vi "Do_ADAM_channel.vi"(4 "Scan Period":dbl format="%.2f", 5 "Previous Scan Value":dbl format="%.2f", 6 "Present scan array":dbl[](array[numeric]) format="%.2f", 7 "Value to Output":dbl format="%.2f", 8 "Ch Description":T1 {"Duty" format="%.0b"; "D" format="%#_5g"; "C" format="%#_5g"; "B" format="%#_5g"; "A" format="%#_5g"}, 9 "Ch names":string[](array[string])) -> (0 "Scan comment":string, 1 "Output":dbl format="%.3f")   [LabVIEW 2012]
uses:
  ADAM Client/Sub VIs/ADAM Controls/Ch_description_ADAM.ctl
  ADAM Client/Sub VIs/ADAM Controls/Module_type_ADAM.ctl
  ADAM Client/Sub VIs/ADAM Controls/Function_ADAM.ctl
  ADAM Client/Sub VIs/ADAM Controls/Channel_State.ctl
  ADAM Client/Sub VIs/ADAM Controls/Calib_type_ADAM.ctl
  ADAM Client/Sub VIs/ADAM Controls/Address.ctl
  ADAM Serial/Instrument drivers/Arduino/ctls_and_globals/Arduino tx msg cluster.ctl
  ADAM Client/Sub VIs/ADAM Controls/Remember_value_mode.ctl
  ADAM Client/Sub VIs/ADAM Controls/Search_mode.ctl
  Anemometry/Anemometry Sub Vis/Controls/In_Range.ctl
  Anemometry/Anemometry Sub Vis/Globals/Gas_management_global.vi
  ADAM_Global.vi
  Anemometry/Anemometry Sub Vis/Globals/Constants_global.vi
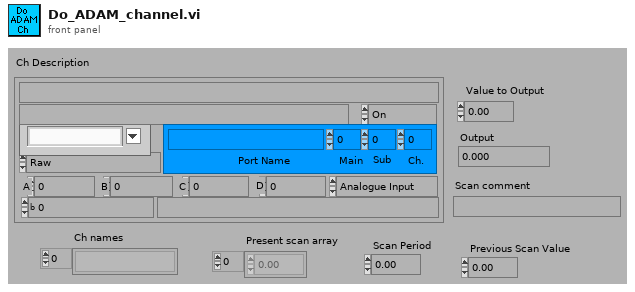
[diagram p1: front panel]
types:
  T1 = typedef "Ch_description_ADAM.ctl" = cluster{"Ch Name":string, "Type":T2, "Function":T3, "Ch State":T4, "Calibration type":T5, "A":dbl, "B":dbl, "C":dbl, "D":dbl, "Comments":string, "Address":T6, "String":string, "Duty":u16}
  T2 = typedef "Module_type_ADAM.ctl" = string
  T3 = typedef "Function_ADAM.ctl" = enum16{"Analogue Input", "Digital Input", "Event counter", "Event rate", "Analogue Output", "Digital Output", "Relay Output"}
  T4 = typedef "Channel_State.ctl" = enum16{"On", "Off", "Always On", "Always Off"}
  T5 = typedef "Calib_type_ADAM.ctl" = enum16{"Raw", "Bx + A", "Cx^2 + Bx + A", "Dx^3 + Cx^2 + Bx + A", "In Band", "Hi-Tec Q", "Hi-Tec M_dot", "Text"}
  T6 = typedef "Address.ctl" = cluster{"Main":i32, "Ch.":i32, "Sub":i32, "Port Name":string}
  T7 = typedef "Remember_value_mode.ctl" = enum16{"Read only", "Read and Write"}
  T8 = typedef "Search_mode.ctl" = enum16{"Between times", "All Times"}
  T9 = typedef "In_Range.ctl" = enum16{"%", "±", "% & ±"}
  T10 = typedef "Arduino tx msg cluster.ctl" = cluster{"dest":u8, "A/D":string, "R/W":string, "chan":u8, "val (float)":sgl}
  T11 = typedef "Valco_valve_ph.ctl" = u16
  T12 = cluster{"Centre Times":dbl[], "Output array":dbl[]}
  T13 = cluster{"Centre Times":dbl[], "Output array":dbl[]}[]
  T14 = typedef "LVDateTimeRec.ctl" = cluster{"fractional second":dbl, "second":i32, "minute":i32, "hour":i32, "day of month":i32, "month":i32, "year":i32, "day of week":i32, "day of year":i32, "DST":i32}
  T15 = typedef "Client_State_Cluster.ctl" = cluster{"Client Name":string, "Traverse level State":T16, "People to Email":string[], "Next Contact Time":dbl}
  T16 = typedef "Traverse_Level_State.ctl" = enum16{"Running", "Complete"}
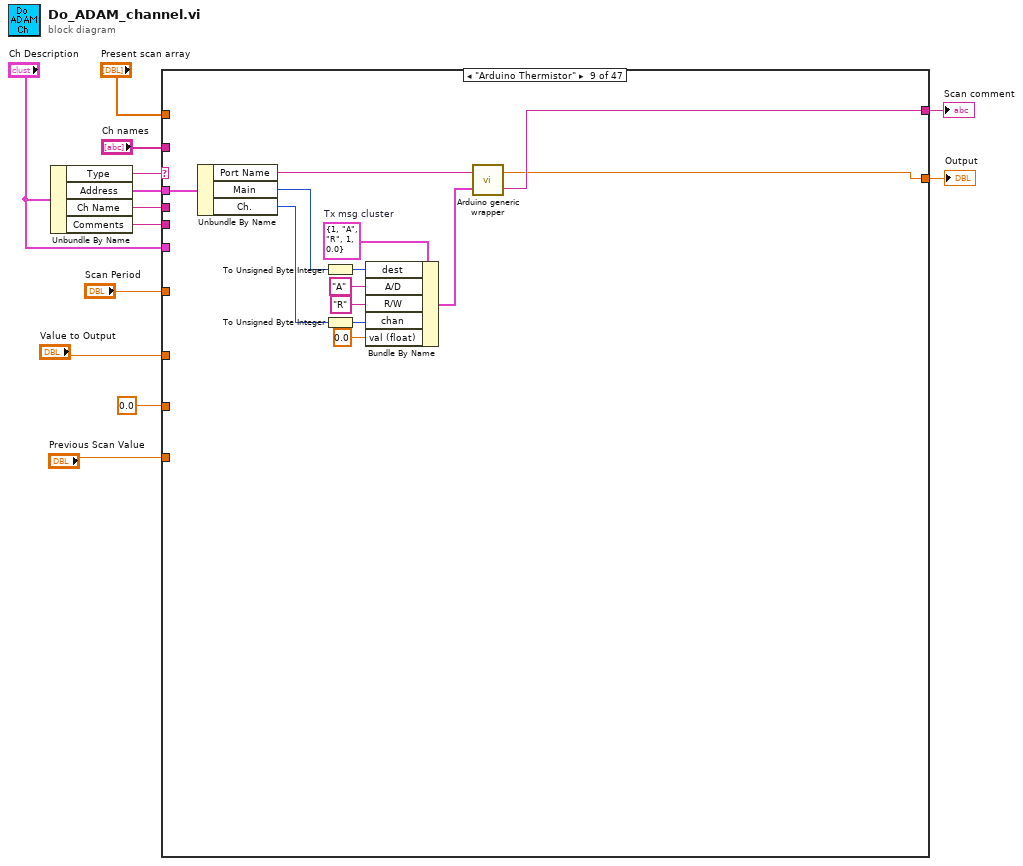
[diagram p0: block diagram]
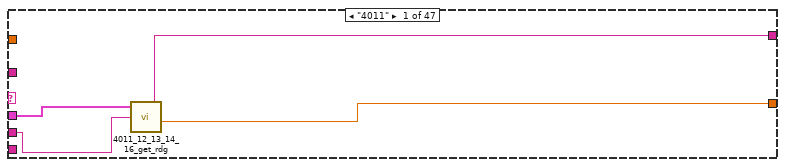
[diagram p2: hidden frame]
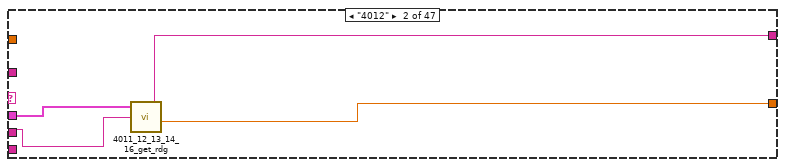
[diagram p3: hidden frame]
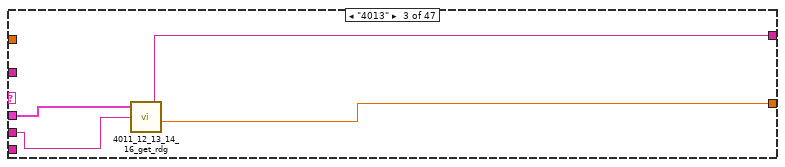
[diagram p4: hidden frame]
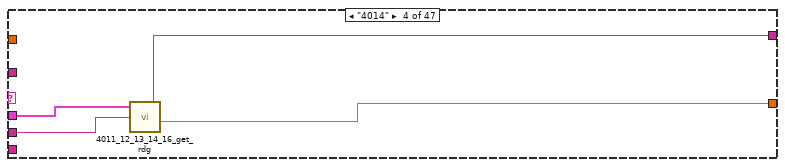
[diagram p5: hidden frame]
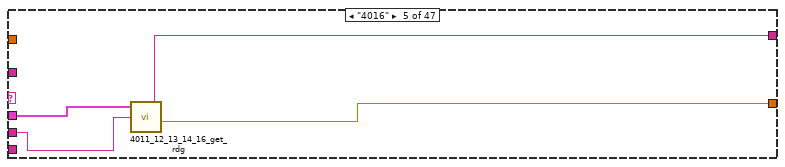
[diagram p6: hidden frame]
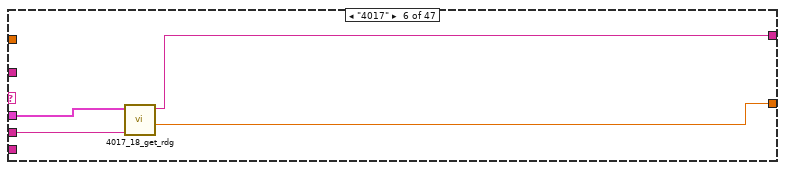
[diagram p7: hidden frame]
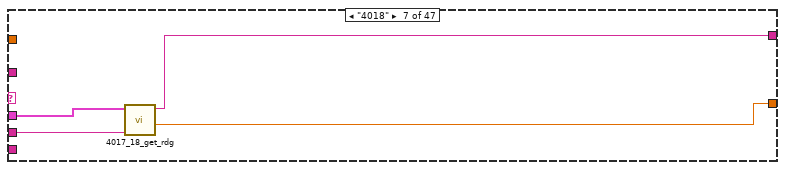
[diagram p8: hidden frame]
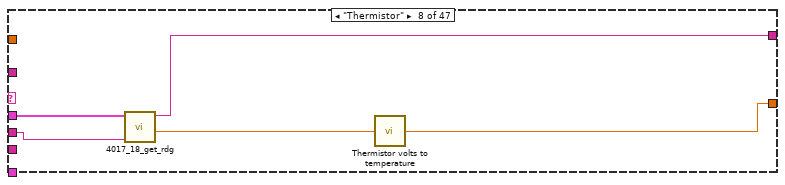
[diagram p9: hidden frame]
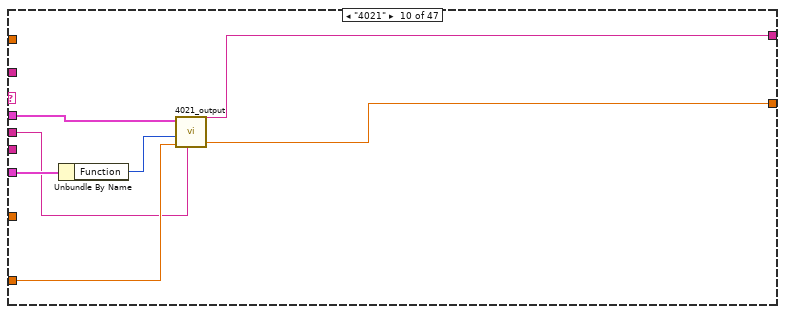
[diagram p10: hidden frame]
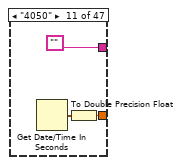
[diagram p11: hidden frame]
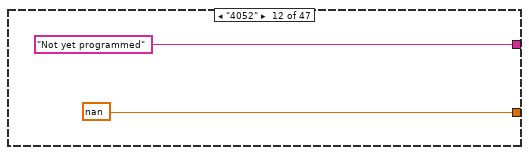
[diagram p12: hidden frame]
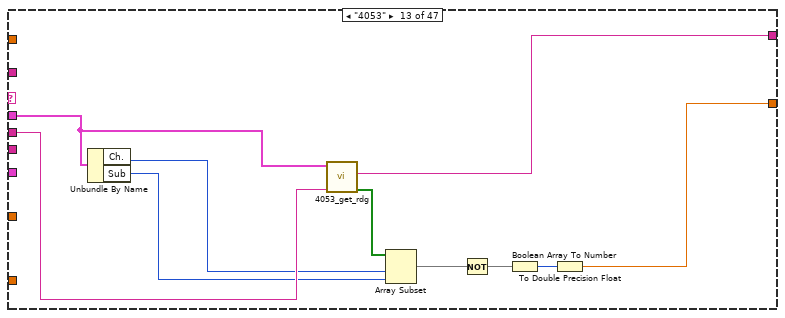
[diagram p13: hidden frame]
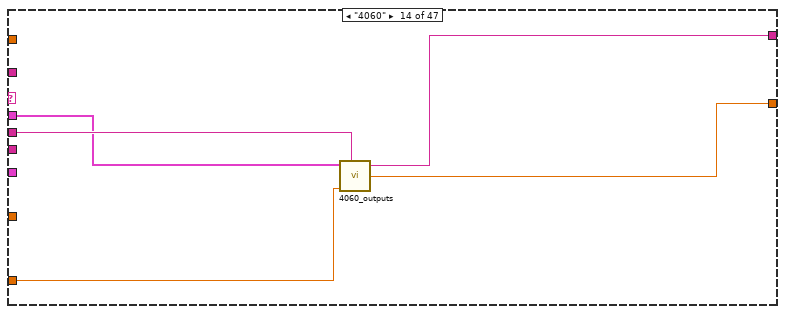
[diagram p14: hidden frame]
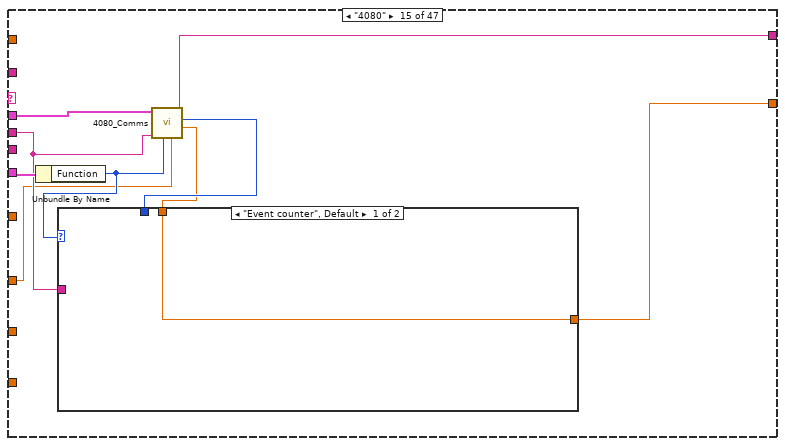
[diagram p15: hidden frame]
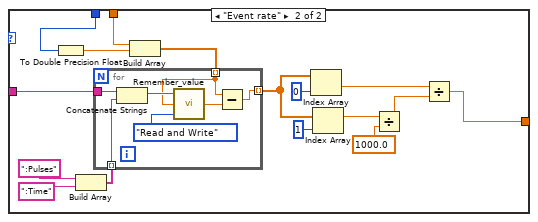
[diagram p16: hidden frame]
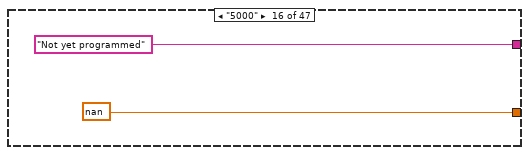
[diagram p17: hidden frame]
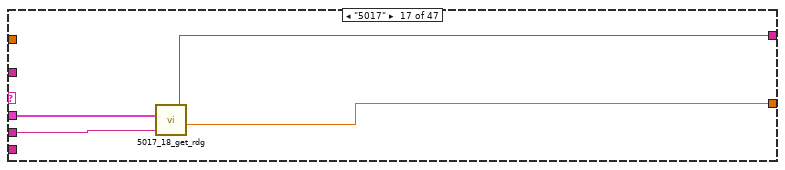
[diagram p18: hidden frame]
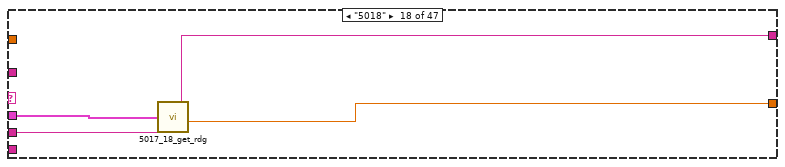
[diagram p19: hidden frame]
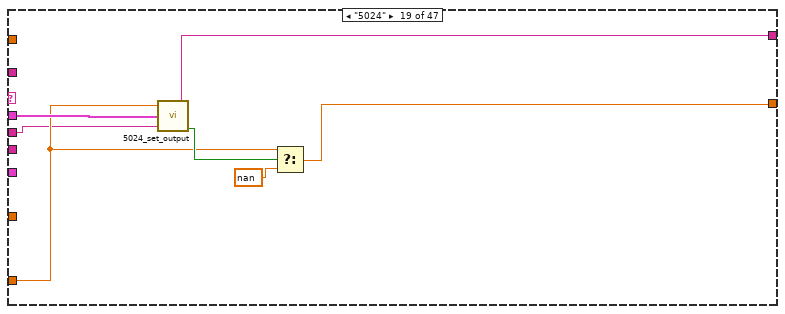
[diagram p20: hidden frame]
diagram:
  n1 = Unbundle By Name("Ch Description") -> ("Type"=w11:T2, "Address"=w10:T6, "Ch Name"=w2:string, "Comments"=w7:string)
  n2 = case shown="\"Arduino Thermistor\"" w11 {
    tunnel: [w16 w20 w24 w28 w32 w36 w40 w42 w47 w65 w68 nan w75 w84 w93 nan w123 w127 w132 w138 w146 w167 w189 w208 nan w276 w278 w294 w317 w356 nan w368 w399 w404 w405 w517 w951 w953 w957 w962 w974 w1008 w1034 w1044 w1049 w1059 0.0 ("Output")] -> w8
    tunnel: [w17 w21 w25 w29 w33 w37 w41 w46 w48 w66 "" "Not yet programmed" w80 w85 w95 "Not yet programmed" w124 w128 w135 w139 w145 w168 w190 w210 "Not yet programmed" w275 w279 w293 w309 w357 "Not yet programmed" w367 w400 w403 w426 w516 "" "" w958 "" "" w997 "" w1045 w1048 "Crazy time based random number!" "Warning; unmatched case in Do_ADAM_channel" ("Status note")] -> w5
    tunnel: w10 -> [w14 w18 w22 w26 w30 w34 w38 w44 w59 w60 _ _ w72 w83 w87 _ w125 w129 w136 w140 w144 w169 w191 w212 _ w273 w277 w296 w314 w362 _ _ w398 w401 _ w508 _ _ _ _ _ _ w1043 w1047 _ _ _]
    tunnel: "Ch Description" -> [_ _ _ _ _ _ _ _ _ w64 _ _ _ _ w94 _ _ _ _ _ w143 w166 w188 w211 _ _ _ _ _ _ _ w373 _ _ w431 w510 _ w954 w959 _ _ _ _ _ w1050 _ _]
    tunnel: w2 -> [w15 w19 w23 w27 w31 w35 w39 w45 _ w61 _ _ w81 w86 w90 _ w122 w126 w130 w137 w141 w163 w185 w209 _ w274 _ w295 w310 w361 _ _ _ w402 _ w513 _ _ _ _ w970 w1004 _ w1046 _ _ _]
    tunnel: "Ch names" -> [_ _ _ _ _ _ _ _ _ _ _ _ _ _ _ _ _ _ _ _ _ _ _ _ _ _ _ _ _ _ _ w374 _ _ w430 w515 _ _ w960 _ _ _ _ _ _ _ _]
    tunnel: "Present scan array" -> [_ _ _ _ _ _ _ _ _ _ _ _ _ _ _ _ _ _ _ _ _ _ _ _ _ _ _ _ _ _ _ w371 _ _ w428 w514 _ _ w961 _ _ _ _ _ _ _ _]
    tunnel: w7 -> [_ _ _ _ _ _ _ _ _ _ _ _ _ _ _ _ _ _ _ _ _ _ _ _ _ _ _ _ _ _ _ w366 _ _ w432 _ _ _ _ _ _ _ _ _ _ _ _]
    tunnel: "Value to Output" -> [_ _ _ _ _ _ _ _ _ w62 _ _ _ w82 w88 _ _ _ w131 _ w142 w164 w186 w207 _ _ _ w292 w318 _ _ w372 _ _ _ _ _ _ _ _ _ _ w1038 _ _ _ _]
    tunnel: "Scan Period" -> [_ _ _ _ _ _ _ _ _ _ _ _ _ _ _ _ _ _ _ _ _ _ _ _ _ _ _ _ _ _ _ w369 _ _ _ w512 _ _ _ _ _ _ _ _ _ _ _]
    tunnel: "Previous Scan Value" -> [_ _ _ _ _ _ _ _ _ _ _ _ _ _ _ _ _ _ _ _ _ _ _ _ _ _ _ _ _ _ _ w370 _ _ w406 w511 w951 _ _ w962 _ _ _ _ _ _ _]
    tunnel: 0.0 -> [_ _ _ _ _ _ _ _ _ _ _ _ _ _ _ _ _ _ _ _ _ _ _ _ _ _ _ _ _ _ _ _ _ _ _ w509 _ _ _ _ _ _ _ _ _ _ _]
    frame "4011" {
      n3 = call "4011_12_13_14_16_get_rdg.vi"("Address"=w14, "Channel Name"=w15) -> ("Comment"=w17:string, "Reading"=w16:dbl)  [unwired: 1 in, 2 out]
    }
    frame "4012" {
      n4 = call "4011_12_13_14_16_get_rdg.vi"("Address"=w18, "Channel Name"=w19) -> ("Comment"=w21:string, "Reading"=w20:dbl)  [unwired: 1 in, 2 out]
    }
    frame "4013" {
      n5 = call "4011_12_13_14_16_get_rdg.vi"("Address"=w22, "Channel Name"=w23) -> ("Comment"=w25:string, "Reading"=w24:dbl)  [unwired: 1 in, 2 out]
    }
    frame "4014" {
      n6 = call "4011_12_13_14_16_get_rdg.vi"("Address"=w26, "Channel Name"=w27) -> ("Comment"=w29:string, "Reading"=w28:dbl)  [unwired: 1 in, 2 out]
    }
    frame "4016" {
      n7 = call "4011_12_13_14_16_get_rdg.vi"("Address"=w30, "Channel Name"=w31) -> ("Comment"=w33:string, "Reading"=w32:dbl)  [unwired: 1 in, 2 out]
    }
    frame "4017" {
      n8 = call "4017_18_get_rdg.vi"("Channel Name"=w35, "Address"=w34) -> ("Reading"=w36:dbl, "Comment"=w37:string)  [unwired: 2 in, 2 out]
    }
    frame "4018" {
      n9 = call "4017_18_get_rdg.vi"("Channel Name"=w39, "Address"=w38) -> ("Reading"=w40:dbl, "Comment"=w41:string)  [unwired: 2 in, 2 out]
    }
    frame "Thermistor" {
      n10 = call "4017_18_get_rdg.vi"("Channel Name"=w45, "Address"=w44) -> ("Reading"=w43:dbl, "Comment"=w46:string)  [unwired: 2 in, 2 out]
      n11 = call "Thermistor volts to temperature.vi"("V2 (V)"=w43) -> ("Temperature (degC)"=w42:dbl)
    }
    frame "Arduino Thermistor" {
      w53 = T10 {"dest"=1, "A/D"="A", "R/W"="R", "chan"=1, "val (float)"=0.0}  # Tx msg cluster
      n12 = Unbundle By Name(w59) -> ("Port Name"=w50:string, "Main"=w51:i32, "Ch."=w52:i32)
      n13 = To Unsigned Byte Integer(number=w51) -> (unsigned 8bit integer=w58:u8)
      n14 = To Unsigned Byte Integer(number=w52) -> (unsigned 8bit integer=w56:u8)
      n15 = Bundle By Name(cluster=w53, "dest"=w58, "A/D"="A", "R/W"="R", "chan"=w56, "val (float)"=sgl 0.0) -> (w49:T10)
      n16 = call "Arduino generic wrapper.vi"("Tx msg cluster"=w49, "Port name"=w50) -> ("Scan comment"=w48:string, "Output"=w47:dbl)
    }
    frame "4021" {
      n17 = Unbundle By Name(w64) -> ("Function"=w63:T3)
      n18 = call "4021_output.vi"("Address"=w60, "Function"=w63, "Set to:"=w62, "Channel Name"=w61) -> ("Comment"=w66:string, "Reading"=w65:dbl)  [unwired: 1 in, 1 out]
    }
    frame "4050" {
      n19 = Get Date/Time In Seconds() -> (seconds since 1Jan1904=w67:timestamp)
      n20 = To Double Precision Float(number=w67) -> (double precision float=w68:dbl)
    }
    frame "4052" {
    }
    frame "4053" {
      n21 = Unbundle By Name(w72) -> ("Ch."=w73:i32, "Sub"=w79:i32)
      n22 = call "4053_get_rdg.vi"("Channel Name"=w81, "Address"=w72) -> ("Boolean array"=w78:bool[], "Comment"=w80:string)  [unwired: 2 in, 2 out]
      n23 = Array Subset(array=w78, index=w73, length=w79) -> (w77:bool[])
      n24 = Not(x=w77) -> (.not. x?=w74:bool[])
      n25 = Boolean Array To Number(Boolean array=w74) -> (number=w76:u32)
      n26 = To Double Precision Float(number=w76) -> (double precision float=w75:dbl)
    }
    frame "4060" {
      n27 = call "4060_outputs.vi"("Address"=w83, "Value to Output"=w82, "Channel Name"=w86) -> ("Comment"=w85:string, "Reading"=w84:dbl)  [unwired: 2 in, 1 out]
    }
    frame "4080" {
      n28 = Unbundle By Name(w94) -> ("Function"=w89:T3)
      n29 = call "4080_Comms.vi"("Value to display"=w88, "Function"=w89, "Channel Name"=w90, "Address"=w87) -> ("Reading"=w91:dbl, "millisecond timer value"=w92:u32, "Comment"=w95:string)  [unwired: 2 in, 1 out]
      n30 = case shown="\"Event counter\", Default" w89 {
        tunnel: w90 -> [_ w112]
        tunnel: w92 -> [_ w105]
        tunnel: [w96 w97] -> w93
        tunnel: w91 -> [w96 w106]
        frame "Event counter", Default {
        }
        frame "Event rate" {
          n31 = To Double Precision Float(number=w105) -> (double precision float=w104:dbl)
          n32 = Build Array(":Pulses", ":Time") -> (w107:string[])
          n33 = Build Array(w106, w104) -> (w103:dbl[])
          n34 = for {
            tunnel: w112 -> [w116]
            tunnel: [w117] -> w100 mode=indexing
            tunnel: w107 -> [w114] mode=indexing
            tunnel: w103 -> [w113] mode=indexing
            n35 = Concatenate Strings(w116, w114) -> (w115:string)
            n36 = call "Remember_value.vi"("Mode"=Remember_value_mode."Read and Write", "Input Value"=w113, "Ch name"=w115) -> ("Output Value"=w118:dbl)
            n37 = Subtract(x=w113, y=w118) -> (x-y=w117:dbl)
          }
          n38 = Index Array(array=w100, index=0) -> (element=w98:dbl)
          n39 = Index Array(array=w100, index=1) -> (element=w99:dbl)
          n40 = Divide(x=w99, y=1000.0) -> (x/y=w110:dbl)
          n41 = Divide(x=w98, y=w110) -> (x/y=w97:dbl)
        }
      }
    }
    frame "5000" {
    }
    frame "5017" {
      n42 = call "5017_18_get_rdg.vi"("Address (all reqd.)"=w125, "Channel Name"=w122) -> ("Comment"=w124:string, "Reading"=w123:dbl)  [unwired: 3 out]
    }
    frame "5018" {
      n43 = call "5017_18_get_rdg.vi"("Address (all reqd.)"=w129, "Channel Name"=w126) -> ("Comment"=w128:string, "Reading"=w127:dbl)  [unwired: 3 out]
    }
    frame "5024" {
      n44 = call "5024_set_output.vi"("Set to:"=w131, "Address (all reqd.)"=w136, "Channel Name"=w130) -> ("Comment"=w135:string, "Good Reply"=w133:bool)  [unwired: 2 out]
      n45 = Select(t=w131, s=w133, f=nan) -> (s? t:f=w132:dbl)
    }
    frame "5051" {
      n46 = call "5051_56_get_inputs.vi"("Address (Main, Sub reqd.)"=w140, "Channel Name"=w137) -> ("Comment"=w139:string, "Single output"=w138:dbl)  [unwired: 3 out]
    }
    frame "5056" {
      n47 = Unbundle By Name(w143) -> ("Function"=w147:T3)
      n48 = case shown="\"Digital Input\"" w147 {
        tunnel: w144 -> [_ w153 w162]
        tunnel: ["This function is not available" w154 w160] -> w145
        tunnel: [nan ("A") w151 w157] -> w146
        tunnel: w142 -> [_ _ w156]
        tunnel: w141 -> [_ w150 w155]
        frame "Analogue Input", Default {
        }
        frame "Digital Input" {
          # "Readback value"
          n49 = call "5060_check_outputs.vi"("Address (Main, Sub reqd.)"=w153, "Channel Name"=w150) -> ("Comment"=w154:string, "Single Channel"=w152:i16)  [unwired: 3 out]
          n50 = To Double Precision Float(number=w152) -> (double precision float=w151:dbl)
        }
        frame "Relay Output" {
          # "Sets single o/p channel"
          n51 = Greater Than 0?(x=w156) -> (x > 0?=w161:bool)
          n52 = call "5056_60_set_single_output.vi"("Channel Name"=w155, "Address (all reqd.)"=w162, "Set state:"=w161) -> ("Comment"=w160:string, "Good Reply"=w159:bool)  [unwired: 2 out]
          n53 = Select(t=w156, s=w159, f=nan) -> (s? t:f=w157:dbl)
        }
      }
    }
    frame "5060" {
      n54 = Unbundle By Name(w166) -> ("Function"=w165:T3)
      n55 = case shown="\"Relay Output\"" w165 {
        tunnel: w169 -> [_ w175 w184]
        tunnel: ["This function is not available" w176 w182] -> w168
        tunnel: [nan ("A") w173 w179] -> w167
        tunnel: w164 -> [_ _ w178]
        tunnel: w163 -> [_ w172 w177]
        frame "Analogue Input", Default {
        }
        frame "Digital Input" {
          # "Readback value"
          n56 = call "5060_check_outputs.vi"("Address (Main, Sub reqd.)"=w175, "Channel Name"=w172) -> ("Comment"=w176:string, "Single Channel"=w174:i16)  [unwired: 3 out]
          n57 = To Double Precision Float(number=w174) -> (double precision float=w173:dbl)
        }
        frame "Relay Output" {
          # "Sets single o/p channel"
          n58 = Greater Than 0?(x=w178) -> (x > 0?=w183:bool)
          n59 = call "5056_60_set_single_output.vi"("Channel Name"=w177, "Address (all reqd.)"=w184, "Set state:"=w183) -> ("Comment"=w182:string, "Good Reply"=w181:bool)  [unwired: 2 out]
          n60 = Select(t=w178, s=w181, f=nan) -> (s? t:f=w179:dbl)
        }
      }
    }
    frame "6060" {
      n61 = Unbundle By Name(w188) -> ("Function"=w187:T3)
      n62 = case shown="\"Digital Input\"" w187 {
        tunnel: w191 -> [_ w197 w206]
        tunnel: ["This function is not available" w198 w204] -> w190
        tunnel: [nan ("A") w195 w201] -> w189
        tunnel: w186 -> [_ _ w200]
        tunnel: w185 -> [_ w194 w199]
        frame "Analogue Input", Default {
        }
        frame "Digital Input" {
          n63 = call "6060_read_all_I-O.vi"("Address (Main, Sub reqd.)"=w197, "Channel Name"=w194) -> ("Comment"=w198:string, "Single Input Channel"=w196:i16)  [unwired: 3 out]
          n64 = To Double Precision Float(number=w196) -> (double precision float=w195:dbl)
        }
        frame "Relay Output" {
          # "Sets single o/p channel"
          n65 = Greater Than 0?(x=w200) -> (x > 0?=w205:bool)
          n66 = call "6060_set_single_output.vi"("Channel Name"=w199, "Address (Main, Ch requd.)"=w206, "Set state:"=w205) -> ("Comment"=w204:string, "Good Reply"=w203:bool)  [unwired: 2 out]
          n67 = Select(t=w200, s=w203, f=nan) -> (s? t:f=w201:dbl)
        }
      }
    }
    frame "Tracker" {
      n68 = while {
        tunnel: w212 -> [w236]
        tunnel: w211 -> [w235]
        tunnel: [w229] -> w210
        tunnel: w209 -> [w228]
        tunnel: [w222] -> w208
        tunnel: w207 -> [w221]
        i -> [w218]
        stop <- w215 continue-if-true
        n69 = Unbundle By Name(w235) -> ("Function"=w234:T3)
        n70 = Unbundle By Name(w236) -> ("Port Name"=w233:string, "Ch."=w224:i32, "Main"=w232:i32, "Sub"=w231:i32)
        n71 = case shown="\"Analogue Output\"" w234 {
          tunnel: [enum16{"Set", "Read"}."Set" ("Set") enum16{"Set", "Read"}."Set" ("Set") enum16{"Set", "Read"}."Set" ("Set") enum16{"Set", "Read"}."Set" ("Set") enum16{"Set", "Read"}."Set" ("Set") enum16{"Set", "Read"}."Read" ("Set") enum16{"Set", "Read"}."Read" ("Set")] -> w219
          tunnel: [enum16{"Logic", "Analogue"}."Analogue" ("Analogue") enum16{"Logic", "Analogue"}."Logic" ("Analogue") enum16{"Logic", "Analogue"}."Logic" ("Analogue") enum16{"Logic", "Analogue"}."Logic" ("Analogue") enum16{"Logic", "Analogue"}."Logic" ("Analogue") enum16{"Logic", "Analogue"}."Logic" ("Analogue") enum16{"Logic", "Analogue"}."Analogue" ("Analogue")] -> w230
          frame "Analogue Output" {
          }
          frame "Digital Output" {
          }
          frame "Relay Output" {
          }
          frame "Event rate" {
          }
          frame "Event counter" {
          }
          frame "Digital Input" {
          }
          frame "Analogue Input" {
          }
        }
        n72 = call "TalkTracker.vi"("PORT NAME"=w233, "Set"=w219, "Channel Name"=w228, "Value to set"=w221, "MODULE ADDRESS"=w232, "LOCATION"=w224, "NO. LOCATIONS"=w231, "Analogue"=w230) -> ("Response"=w226:string, "Good Set?"=w213:bool, "Comment out"=w229:string)  [unwired: 1 in, 4 out]
        n73 = Match Pattern(string=w226, regular expression="\r\n") -> (before substring=w225:string)  [unwired: 4 out]
        n74 = case shown="\"Set\"" w219 {
          tunnel: w225 -> [_ w248]
          tunnel: [w240 w247] -> w223
          tunnel: w221 -> [w242 _]
          tunnel: nan ("Reading") -> [w241 w246]
          tunnel: [w239 w244] -> w216
          tunnel: [0 ("y") 1 ("y")] -> w214
          tunnel: w213 -> [w237 _]
          frame "Set" {
            n75 = Not(x=w237) -> (.not. x?=w239:bool)
            n76 = Select(t=w242, s=w237, f=w241) -> (s? t:f=w240:dbl)
          }
          frame "Read" {
            n77 = String Length(string=w248) -> (length=w250:i32)
            n78 = Fract/Exp String To Number(string=w248, default (0 dbl)=w246) -> (offset past number=w251:i32, number=w249:dbl)  [unwired: 2 out]
            n79 = Equal?(x=w250, y=w251) -> (x = y?=w245:bool)
            n80 = Not(x=w245) -> (.not. x?=w244:bool)
            n81 = Select(t=w249, s=w245, f=w246) -> (s? t:f=w247:dbl)
          }
        }
        n82 = case shown="0, Default" w224 {
          tunnel: w223 -> [w252 w255]
          tunnel: [w252 w253] -> w222
          frame 0, Default {
          }
          frame 283 {
            n83 = Equal To 0?(x=w255) -> (x = 0?=w256:bool)
            n84 = Select(t=nan ("Reading"), s=w256, f=w255) -> (s? t:f=w253:dbl)
          }
        }
        n85 = Less?(x=w218, y=w214) -> (x < y?=w217:bool)
        n86 = And(x=w216, y=w217) -> (x .and. y?=w215:bool)
      }
    }
    frame "WEST" {
    }
    frame "GILL" {
      n87 = call "Gill_get_rdg.vi"("Channel Name"=w274, "Address"=w273) -> ("Output"=w276:dbl, "Status note"=w275:string)  [unwired: 2 in, 2 out]
    }
    frame "ClimatronicsUDP" {
      n88 = call "ClimatronicsUDP_get_rdg.vi"("Address"=w277) -> ("Output"=w278:dbl, "Status note"=w279:string)  [unwired: 5 in]
    }
    frame "JEM" {
      n89 = Unbundle By Name(w296) -> ("Main"=w282:i32, "Ch."=w281:i32, "Port Name"=w291:string)
      n90 = case shown="0, Default" w281 {
        tunnel: [i16[] [-3, -2, -1, 0, 14, 29, 43, 57, 71, 86, 100] i16[] [0, 20, 40, 60, 80, 100, 120]] -> w285
        tunnel: [u8[] [10, 50, 80, 100, 120, 140, 160, 180, 200, 220, 240] u8[] [20, 50, 90, 130, 160, 200, 230]] -> w286
        frame 0, Default {
        }
        frame 1 {
        }
      }
      n91 = Add(x=w282, y=w281) -> (x+y=w280:i32)
      n92 = Threshold 1D Array(2:w292, 3:w285) -> (0:w288:dbl)  [unwired: 1 out]
      n93 = Round To Nearest(number=w288) -> (nearest integer value=w289:dbl)
      n94 = To Long Integer(number=w289) -> (32bit integer=w287:i32)
      n95 = Index Array(array=w286, index=w287) -> (element=w284:u8)
      n96 = call "DMX.vi"("Port Name"=w291, "DMX channel no."=w280, "Set value:"=w284, "Channel Name"=w295) -> ("error"=w290:bool)  [unwired: 2 out]
      n97 = Index Array(array=w285, index=w287) -> (element=w283:i16)
      n98 = case shown="False" w290 {
        tunnel: [w297 nan] -> w294
        tunnel: ["" "Comms Error"] -> w293
        tunnel: w283 -> [w299 _]
        frame False {
          n99 = To Double Precision Float(number=w299) -> (double precision float=w297:dbl)
        }
        frame True {
        }
      }
    }
    frame "VICI" {
      n100 = To Long Integer(number=w318) -> (32bit integer=w313:i32)
      n101 = Unbundle By Name(w314) -> ("Port Name"=w316:string, "Ch."=w315:i32)
      n102 = call "Valco_Valve_Position.vi"("Channel Name"=w310, "Valve Number"=w315, "Port Name"=w316, "Requested Posn."=w313) -> ("Error Message"=w308:string, "Achieved Posn."=w311:T11)  [unwired: 2 out]
      n103 = Empty String/Path?(string/path=w308) -> ()  [unwired: 1 out]
      n104 = case shown="True" TRUE {
        tunnel: w314 -> [w325 _]
        tunnel: w313 -> [w324 _]
        tunnel: [w323 w355] -> w312
        tunnel: w311 -> [_ w355]
        tunnel: w310 -> [w322 _]
        tunnel: [w321 w354] -> w309
        tunnel: w308 -> [_ w354]
        tunnel: w308 -> [w320 _]
        tunnel: "X10" ("Port Name") -> [w319 _]
        frame False {
          n105 = stacked-sequence {
            tunnel: w325 -> [_ _ _ _ _ w346]
            tunnel: w324 -> [_ _ _ _ _ w342]
            tunnel: [_ _ _ _ _ w345] -> w323
            tunnel: w322 -> [_ _ _ _ _ w344]
            tunnel: [_ _ _ _ _ w343] -> w321
            tunnel: w320 -> [_ w331 _ _ _ _]
            tunnel: w319 -> [w326 _ _ w334 _ _]
            frame #0 {
              w328 = 3 items=["-----", "A", "B", "C", "D", "E", "F", "G", "H", "I", "J", "K", "L", "M", "N", "O", "P"] ("House Code")
              n106 = call "X10control.vi"("Port Name"=w326, "Power Request (ON)"=FALSE, "House Code"=w328, "Unit No."=5) -> ()  [unwired: 6 out]
            }
            frame #1 {
              n107 = call "Server_Emails.vi"("Message"=w331, "Contact All clients?"=TRUE, "Subject"="Powering Down FID Valve" ("Error Type")) -> ()  [unwired: 2 in, 3 out]
            }
            frame #2 {
              n108 = Wait (ms)(milliseconds to wait=u32 20000) -> ()  [unwired: 1 out]
            }
            frame #3 {
              w336 = 3 items=["-----", "A", "B", "C", "D", "E", "F", "G", "H", "I", "J", "K", "L", "M", "N", "O", "P"] ("House Code")
              n109 = call "X10control.vi"("Port Name"=w334, "Power Request (ON)"=TRUE, "House Code"=w336, "Unit No."=5) -> ()  [unwired: 6 out]
            }
            frame #4 {
              n110 = Wait (ms)(milliseconds to wait=u32 5000) -> ()  [unwired: 1 out]
            }
            frame #5 {
              n111 = Build Array(1 ("element"), 2 ("element"), w342) -> (w339:i32[])
              n112 = for {
                tunnel: w346 -> [w351]
                tunnel: [w350] -> w345
                tunnel: w344 -> [w349]
                tunnel: [w348] -> w343
                tunnel: w339 -> [w347] mode=indexing
                n113 = Unbundle By Name(w351) -> ("Port Name"=w352:string, "Ch."=w353:i32)
                n114 = call "Valco_Valve_Position.vi"("Channel Name"=w349, "Valve Number"=w353, "Port Name"=w352, "Requested Posn."=w347) -> ("Error Message"=w348:string, "Achieved Posn."=w350:T11)  [unwired: 2 out]
              }
            }
          }
        }
        frame True {
        }
      }
      n115 = To Double Precision Float(number=w312) -> (double precision float=w317:dbl)
    }
    frame "Vaisala" {
      n116 = Unbundle By Name(w362) -> ("Main"=w358:i32, "Ch."=w359:i32, "Port Name"=w360:string)
      n117 = call "HMP231.vi"("Channel Name"=w361, "Port Name"=w360, "Channel"=w359, "Address"=w358) -> ("Output"=w356:dbl, "Status note"=w357:string)  [unwired: 2 out]
    }
    frame "DRUCK" {
    }
    frame "Run VI Named:" {
      n118 = Current VI's Path() -> (path=w383:path)
      n119 = Strip Path(path=w383) -> (stripped path=w384:path)  [unwired: 1 out]
      n120 = call <vilib>:"Trim Whitespace.vi"("string"=w366) -> ("trimmed string"=w365:string)  [unwired: 1 in]
      n121 = Strip Path(path=w384) -> (stripped path=w385:path)  [unwired: 1 out]
      n122 = Build Path(base path=w385, name or relative path="Run_vi_named") -> (appended path=w387:path)
      n123 = Build Path(base path=w387, name or relative path=w365) -> (appended path=w382:path)
      n124 = Open VI Reference(type specifier VI Refnum (for type only)=refnum<vi> refnum, vi path=w382) -> (vi reference=w378:refnum<vi>, error out=w377:errorcluster)  [unwired: 1 in, 3 out]
      n125 = property class="VI Interface Type 0"(reference=w378, error in=w377) -> (reference out=w380:refnum<vi>, error out=w379:errorcluster, "Front Panel Window:Open"=w381:bool)
      n126 = case shown="False" w381 {
        tunnel: w380 -> [w395 w397]
        tunnel: w379 -> [w394 w396]
        tunnel: [w393 w397] -> w376
        tunnel: [w391 w396] -> w375
        frame False {
          n127 = property class="VI Interface Type 0"(reference=w395, error in=w394, "Front Panel Window:Open"=TRUE) -> (reference out=w393:refnum<vi>, error out=w391:errorcluster)
        }
        frame True {
        }
      }
      n128 = call-by-ref "?"(reference=w376, error in=w375, "Scan Period"=w369, "Previous Scan Value"=w370, "Present scan array"=w371, "Value to Output"=w372, "Ch Description"=w373, "Ch names"=w374) -> (reference out=w389:refnum<vi>, error out=w390:errorcluster, "Scan comment"=w367:string, "Output"=w368:dbl)  [unwired: 2 in]
      n129 = Close Reference(reference=w389, error in (no error)=w390) -> ()  [unwired: 1 out]
    }
    frame "IR2100" {
      n130 = call "IR2100_get_rdg.vi"("Address"=w398) -> ("Comment"=w400:string, "Reading"=w399:dbl)  [unwired: 2 in, 2 out]
    }
    frame "PPT" {
      n131 = call "PPT_get_rdg.vi"("Channel Name"=w402, "Address"=w401) -> ("Reading"=w404:dbl, "Comment"=w403:string)  [unwired: 2 in, 2 out]
    }
    frame "Comparator" {
      # "A Warn if above this value\nB Warn if below this value\nC  Hysteresis margin\nD is the averaging time in minutes\nComments   is Channel name to check"
      n132 = Unbundle By Name(w431) -> ("D"=w414:dbl)
      n133 = Match Pattern(string=w432, regular expression=":::" ("String to match")) -> (before substring=w429:string)  [unwired: 4 out]
      n134 = call "Read_value_of_earlier_Ch.vi"("Desired Ch to Read"=w429, "Ch names"=w430, "Present scan array"=w428) -> ("Value"=w413:dbl, "Scan comment"=w427:string)  [unwired: 1 in]
      n135 = Equal?(x=w406, y=1.0) -> (x = y?=w422:bool)
      n136 = Unbundle By Name(w431) -> ("A"=w425:dbl, "B"=w424:dbl, "C"=w423:dbl)
      n137 = Equal To 0?(x=w414) -> (x = 0?=w412:bool)
      n138 = case shown="True" w422 {
        tunnel: [w438 w443] -> w420
        tunnel: w425 -> [w438 w442]
        tunnel: w424 -> [w437 w441]
        tunnel: [w437 w439] -> w421
        tunnel: w423 -> [_ w440]
        frame False {
        }
        frame True {
          n139 = Subtract(x=w442, y=w440) -> (x-y=w443:dbl)
          n140 = Add(x=w441, y=w440) -> (x+y=w439:dbl)
        }
      }
      n141 = case shown="False" w412 {
        tunnel: [w448 w451] -> w435
        tunnel: w429 -> [w450 _]
        tunnel: [w446 w452] -> w411
        tunnel: w414 -> [w444 _]
        tunnel: w413 -> [_ w452]
        tunnel: w427 -> [w448 w451]
        frame False {
          n142 = Build Array(w450) -> (w445:string[])
          n143 = call "Get_Channel_averages.vi"("Desired Ch Names"=w445, "Averaging time (mins)"=w444) -> ("number"=w447:dbl[])  [unwired: 1 in, 2 out]
          n144 = Index Array(array=w447, index=0) -> (element=w446:dbl)
        }
        frame True {
        }
      }
      n145 = Not(x=w422) -> (.not. x?=w415:bool)
      n146 = In Range and Coerce(upper limit=w420, x=w411, lower limit=w421) -> (In Range?=w416:bool)  [unwired: 1 out]
      n147 = Greater?(x=w411, y=w420) -> (0:w419:bool)
      n148 = Not A Number/Path/Refnum?(number/path/refnum=w411) -> (NaN/Path/Refnum?=w408:bool)
      n149 = Equal?(x=w416, y=w415) -> (x = y?=w410:bool)
      n150 = Or(x=w410, y=w408) -> (x .or. y?=w409:bool)
      n151 = case shown="False" w409 {
        tunnel: w429 -> [w459 _]
        tunnel: w420 -> [w458 _]
        tunnel: w431 -> [w457 _]
        tunnel: w421 -> [w456 _]
        tunnel: w416 -> [w455 _]
        tunnel: w411 -> [w454 _]
        tunnel: w419 -> [w453 _]
        frame False {
          n152 = stacked-sequence {
            seq-local: [w465 _ _ _ _] -> [_ _ _ w506 _]
            seq-local: [_ w485 _ _ _] -> [_ _ _ w503 _]
            seq-local: [w463 _ _ _ _] -> [_ _ _ w499 _]
            tunnel: w459 -> [w467 w493 _ w505 _]
            tunnel: w458 -> [w466 _ _ _ _]
            tunnel: w457 -> [_ _ w498 w507 _]
            tunnel: w456 -> [w464 _ _ _ _]
            tunnel: w455 -> [w462 _ _ _ _]
            tunnel: w454 -> [w461 _ _ _ _]
            tunnel: w453 -> [w460 _ _ _ _]
            frame #0 {
              n153 = case shown="True" w462 {
                tunnel: w467 -> [w472 w483]
                tunnel: w466 -> [_ w476]
                tunnel: [w470 w482] -> w465
                tunnel: w464 -> [_ w475]
                tunnel: ["OK " ""] -> w463
                tunnel: w461 -> [w468 _]
                tunnel: w460 -> [_ w473]
                frame True {
                  n154 = Format Into String(format string="The channel named %s is now  %.3f" ("Format String"), w472, w468) -> (resulting string=w470:string)  [unwired: 2 in, 1 out]
                }
                frame False {
                  n155 = Select(t=w476, s=w473, f=w475) -> (s? t:f=w474:dbl)
                  n156 = Select(t="greater", s=w473, f="less") -> (s? t:f=w478:string)
                  n157 = Format Into String(format string="%s is %s than %.3f" ("Format String"), w483, w478, w474) -> (resulting string=w482:string)  [unwired: 2 in, 1 out]
                }
              }
            }
            frame #1 {
              n158 = Build Array(w493) -> (w492:string[])
              n159 = call "Channel_Names_and_indicies.vi"("All Active Channels"=FALSE, "Desired Ch Names"=w492) -> ("Indicies"=w490:i32[])  [unwired: 1 out]
              n160 = call "Specified_Channels_server.vi"("Mode"=Search_mode."All Times", "Requested channels"=w490) -> ("Output array"=w488:dbl[][], "Centre Times"=w484:dbl[])  [unwired: 3 in, 3 out]
              n161 = Index Array(array=w488, index (row)=0) -> (element=w486:dbl[])  [unwired: 1 in]
              n162 = Bundle("Centre Times"=w484, "Output array"=w486) -> (w489:T12)  [unwired: 1 out]
              n163 = Build Array(w489) -> (w485:T13)
            }
            frame #2 {
              w496 = TRUE  # Contact All clients?
              n164 = Unbundle By Name(w498) -> ("String"=w497:string)
              n165 = call "Get_array_values_fr_String.vi"("String Value"=w497) -> ("String array"=w495:string[])  [unwired: 1 out]
              n166 = call "Client_email_addresses.vi"("Extra People to Email"=w495, "Contact All clients?"=w496) -> ()  [unwired: 1 in]
            }
            frame #3 {
              n167 = Unbundle By Name(w507) -> ("Ch Name"=w500:string)
              n168 = Build Array(w505) -> (w504:string[])
              n169 = Concatenate Strings(w499, w500) -> (w501:string)
              n170 = call "Email_Attachment_Plot.vi"("X axis name"="Time", "XY Graph"=w503, "Series Names"=w504, "message"=w506, "subject ([No Subject])"=w501) -> ()  [unwired: 1 in, 1 out]
            }
            frame #4 {
            }
          }
        }
        frame True {
        }
      }
      n171 = Concatenate Strings(w435, "") -> (w426:string)
      n172 = Select(t=0.0, s=w416, f=1.0) -> (s? t:f=w407:dbl)
      n173 = Select(t=w406, s=w408, f=w407) -> (s? t:f=w405:dbl)
    }
    frame "VIRTUAL" {
      n174 = case shown="\"EnFlo_Tunnel:Inlet:K_Factor\"" w513 {
        tunnel: [w527 w541 w555 w577 w592 w603 w619 w650 w677 w712 w716 w750 w801 w827 w854 w874] -> w517
        tunnel: [w518 w547 w553 w581 w586 w601 w628 "" w681 w706 w722 w747 w800 w826 "" w875] -> w516
        tunnel: w515 -> [w524 w549 w559 w583 w588 w606 w630 w654 w683 w708 w724 w748 w806 w831 _ w877]
        tunnel: w514 -> [w525 w548 w560 w582 w587 w607 w629 w655 w684 w707 w723 w749 w808 w833 _ w876]
        tunnel: w513 -> [w522 _ _ _ _ _ _ _ _ _ _ w736 _ _ w849 _]
        tunnel: w512 -> [w523 _ _ _ _ _ _ _ _ _ _ _ w798 w825 w854 w873]
        tunnel: w511 -> [w526 _ _ _ _ _ _ _ _ _ _ w751 w802 w828 _ w872]
        tunnel: w510 -> [_ _ w551 _ _ _ _ _ _ _ _ w742 _ _ _ _]
        tunnel: w509 -> [_ w540 _ _ _ w600 _ _ _ _ _ _ _ _ _ _]
        tunnel: w508 -> [_ _ _ _ _ _ _ _ _ _ _ _ _ _ _ _]
        frame "GMU:Remaining:", Default {
          n175 = Match Pattern(string=w522, regular expression="GMU:Remaining:" ("String to match")) -> (match substring=w520:string)  [unwired: 4 out]
          n176 = Empty String/Path?(string/path=w520) -> (empty?=w519:bool)
          n177 = case shown="False" w519 {
            tunnel: [w534 nan] -> w527
            tunnel: w526 -> [w533 _]
            tunnel: w525 -> [w532 _]
            tunnel: w524 -> [w531 _]
            tunnel: w523 -> [w530 _]
            tunnel: w522 -> [w529 _]
            tunnel: [w528 w536] -> w518
            frame False {
              n178 = call "Update_Rem_gas.vi"("Scan Period (s)"=w530, "Gas Remaining in"=w533, "Ch name"=w529, "Ch names"=w531, "Present scan array"=w532) -> ("Gas Remaining out"=w534:dbl, "Comments"=w528:string)  [unwired: 1 out]
            }
            frame True {
              n179 = Current VI's Path() -> (path=w538:path)
              n180 = Path To String(path=w538) -> (string=w537:string)
              n181 = Concatenate Strings(" was not matched in ", w537) -> (w536:string)
            }
          }
        }
        frame "GMU:Source:Meas Q" {
          n182 = call "Calculate_Release_Flowrates.vi"("Ch names"=w549, "Units"=enum16{"Q l/min", "M_dot Kg/min"}."Q l/min", "Present scan array"=w548) -> ("Trace"=w545:dbl, "Carrier"=w546:dbl, "Scan comments"=w547:string)
          n183 = Add(x=w546, y=w545) -> (x+y=w542:dbl)
          n184 = Not Equal To 0?(x=w542) -> (x != 0?=w543:bool)
          n185 = Select(t=w542, s=w543, f=w540) -> (s? t:f=w541:dbl)
        }
        frame "GMU:Detector:Strength" {
          n186 = Unbundle By Name(w551) -> ("C"=w550:dbl)
          n187 = call "Read_value_of_earlier_Ch.vi"("Desired Ch to Read"="GMU:Detector:Meas Current", "Ch names"=w559, "Present scan array"=w560) -> ("Value"=w556:dbl, "Scan comment"=w554:string)  [unwired: 1 in]
          n188 = Greater?(x=w556, y=w550) -> (0:w557:bool)
          n189 = case shown="True" w557 {
            tunnel: w551 -> [_ w572]
            tunnel: w556 -> [_ w567]
            tunnel: [100.0 ("Eng Values") w565] -> w555
            tunnel: ["Fault" w568] -> w552
            frame False {
            }
            frame True {
              n190 = Unbundle By Name(w572) -> ("D"=w563:dbl, "A"=w571:dbl, "B"=w570:dbl)
              n191 = Less?(x=w567, y=w563) -> (x < y?=w566:bool)
              n192 = Build Array(w571, w570) -> (w569:dbl[])
              n193 = call "Polynomial_convert.vi"("Calib constants"=w569, "Voltage"=w567) -> ("Eng Values"=w564:dbl)  [unwired: 4 out]
              n194 = case shown="True" w566 {
                tunnel: ["Saturated" ""] -> w568
                tunnel: [100.0 ("Eng Values") w575] -> w565
                tunnel: w564 -> [_ w575]
                frame False {
                }
                frame True {
                }
              }
            }
          }
          n195 = Concatenate Strings(w554, w552) -> (w553:string)
        }
        frame "GMU:Source:Meas M_dot" {
          n196 = call "Calculate_Release_Flowrates.vi"("Ch names"=w583, "Units"=enum16{"Q l/min", "M_dot Kg/min"}."M_dot Kg/min", "Present scan array"=w582) -> ("Trace"=w579:dbl, "Carrier"=w580:dbl, "Scan comments"=w581:string)
          n197 = Add(x=w580, y=w579) -> (x+y=w577:dbl)
        }
        frame "GMU:Source:Meas Density" {
          n198 = Build Array("GMU:Source:Meas M_dot", "GMU:Source:Meas Q") -> (w589:string[])
          n199 = call "Read_Earlier_Channels.vi"("Present scan array"=w587, "Ch names"=w588, "Desired Channels"=w589) -> ("Scan comments"=w586:string, "Index 0"=w585:dbl, "Index 1"=w584:dbl)  [unwired: 3 out]
          n200 = Not Equal To 0?(x=w585) -> (x != 0?=w593:bool)
          n201 = case shown="False" w593 {
            tunnel: w585 -> [_ w597]
            tunnel: w584 -> [_ w596]
            tunnel: [0.0 w595] -> w592
            frame False {
            }
            frame True {
              n202 = Divide(x=w597, y=w596) -> (x/y=w598:dbl)
              n203 = Multiply(x=w598, y=1000.0) -> (x*y=w595:dbl)
            }
          }
        }
        frame "GMU:Source:Meas Den Ratio" {
          n204 = call "Read_value_of_earlier_Ch.vi"("Desired Ch to Read"="GMU:Source:Meas Density", "Ch names"=w606, "Present scan array"=w607) -> ("Value"=w602:dbl, "Scan comment"=w601:string)  [unwired: 1 in]
          n205 = Equal?(x=w602, y=w600) -> (x = y?=w604:bool)
          n206 = case shown="False" w604 {
            tunnel: w602 -> [w609 _]
            tunnel: [w608 w614] -> w603
            tunnel: w600 -> [_ w614]
            frame False {
              n207 = global read "Gas_management_global.vi" "Release temp (deg C)"() -> (w612:dbl)
              n208 = global read "Gas_management_global.vi" "Atmos Pres (mbars)"() -> (w611:dbl)
              n209 = call "Gas_Density.vi"("Pressure (mbars)"=w611, "Temperature (deg C)"=w612, "Gas Name"="Air") -> ("Density Kg/m3"=w610:dbl)
              n210 = Divide(x=w609, y=w610) -> (x/y=w608:dbl)
            }
            frame True {
            }
          }
        }
        frame "GMU:Source:Meas Strength" {
          n211 = call "Calculate_Release_Flowrates.vi"("Ch names"=w630, "Units"=enum16{"Q l/min", "M_dot Kg/min"}."Q l/min", "Present scan array"=w629) -> ("Trace"=w622:dbl, "Carrier"=w623:dbl, "Scan comments"=w628:string)
          n212 = Equal To 0?(x=w623) -> (x = 0?=w625:bool)
          n213 = Equal To 0?(x=w622) -> (x = 0?=w626:bool)
          n214 = And(x=w625, y=w626) -> (x .and. y?=w624:bool)
          n215 = case shown="False" w624 {
            tunnel: w623 -> [w641 _]
            tunnel: w622 -> [w640 _]
            tunnel: [w639 0.0] -> w618
            frame False {
              n216 = Add(x=w641, y=w640) -> (x+y=w644:dbl)
              n217 = Divide(x=w640, y=w644) -> (x/y=w643:dbl)
              n218 = Multiply(x=w643, y=100.0) -> (x*y=w639:dbl)
            }
            frame True {
            }
          }
          n219 = while {
            tunnel: [w632] -> w615
            tunnel: [w633] -> w617
            tunnel: w618 -> [w638]
            shift-left: _ -> [w632]
            shift-left: _ -> [w637]
            shift-right: [w638] -> _
            stop <- FALSE continue-if-true
            w636 = 6.0 ("y")
            n220 = Less?(x=w637, y=w636) -> (x < y?=w635:bool)
            n221 = Less?(x=w632, y=w636) -> (x < y?=w634:bool)
            n222 = Or(x=w635, y=w634) -> (x .or. y?=w633:bool)
          }
          n223 = Greater?(x=w618, y=7.0) -> (0:w616:bool)
          n224 = And(x=w617, y=w616) -> (x .and. y?=w620:bool)
          n225 = Select(t=w615, s=w620, f=w618) -> (s? t:f=w619:dbl)
        }
        frame "EnFlo_Tunnel:Temp:Inlet_Av" {
          w653 = 0.0 ("Value")
          w647 = "EnFlo_Tunnel:Temp:Inlet"
          n226 = String Length(string=w647) -> (length=w648:i32)
          n227 = for {
            tunnel: w655 -> [w661] mode=indexing
            tunnel: w654 -> [w660] mode=indexing
            shift-right: [w668] -> w652
            shift-left: w653 -> [w667]
            shift-right: [w665] -> w651
            shift-left: w653 -> [w666]
            tunnel: w648 -> [w664]
            tunnel: w647 -> [w662]
            tunnel: "EnFlo_Tunnel:Temp:Inlet_Av" -> [w659]
            n228 = String Subset(string=w660, length (rest)=w664) -> (substring=w663:string)  [unwired: 1 out]
            n229 = Equal?(x=w663, y=w662) -> (x = y?=w657:bool)
            n230 = Not Equal?(x=w660, y=w659) -> (x != y?=w658:bool)
            n231 = And(x=w657, y=w658) -> (x .and. y?=w656:bool)
            n232 = case shown="True" w656 {
              tunnel: [w670 w674] -> w668
              tunnel: w667 -> [w670 w675]
              tunnel: w661 -> [_ w673]
              tunnel: w666 -> [w669 w672]
              tunnel: [w669 w671] -> w665
              frame False {
              }
              frame True {
                n233 = Add(x=w673, y=w675) -> (x+y=w674:dbl)
                n234 = Increment(x=w672) -> (x+1=w671:dbl)
              }
            }
          }
          n235 = Divide(x=w652, y=w651) -> (x/y=w650:dbl)
        }
        frame "EnFlo Lab:labstrat1:Av Temp" {
          w680 = 0.0 ("Value")
          n236 = for {
            tunnel: w684 -> [w696]
            tunnel: w683 -> [w695]
            shift-right: [w692] -> w681
            shift-left: "" -> [w693]
            shift-right: [w690] -> w679
            shift-left: w680 -> [w689]
            shift-right: [w686] -> w678
            shift-left: w680 -> [w687]
            tunnel: string[] ["EnFlo Lab:labstrat1:Z=4.5m", "EnFlo Lab:labstrat1:Z=3.5m", "EnFlo Lab:labstrat1:Z=2.5m", "EnFlo Lab:labstrat1:Z=1.5m", "EnFlo Lab:labstrat1:Z=0.5m"] -> [w685] mode=indexing
            n237 = call "Read_value_of_earlier_Ch.vi"("Desired Ch to Read"=w685, "Ch names"=w695, "Present scan array"=w696) -> ("Value"=w688:dbl, "Scan comment"=w694:string)  [unwired: 1 in]
            n238 = Concatenate Strings(w693, w694) -> (w692:string)
            n239 = Not A Number/Path/Refnum?(number/path/refnum=w688) -> (NaN/Path/Refnum?=w691:bool)
            n240 = case shown="True" w691 {
              tunnel: [w700 w703] -> w690
              tunnel: w689 -> [w701 w703]
              tunnel: w688 -> [w699 _]
              tunnel: w687 -> [w698 w702]
              tunnel: [w697 w702] -> w686
              frame False {
                n241 = Add(x=w699, y=w701) -> (x+y=w700:dbl)
                n242 = Increment(x=w698) -> (x+1=w697:dbl)
              }
              frame True {
              }
            }
          }
          n243 = Divide(x=w679, y=w678) -> (x/y=w677:dbl)
        }
        frame "EnFlo Lab:labstrat1:Delta T" {
          n244 = Build Array("EnFlo Lab:labstrat1:Z=4.5m", "EnFlo Lab:labstrat1:Z=0.5m") -> (w711:string[])
          n245 = call "Read_Earlier_Channels.vi"("Present scan array"=w707, "Ch names"=w708, "Desired Channels"=w711) -> ("Scan comments"=w706:string, "Index 0"=w705:dbl, "Index 1"=w704:dbl)  [unwired: 3 out]
          n246 = Subtract(x=w705, y=w704) -> (x-y=w712:dbl)
        }
        frame "EnFlo_Tunnel:Inlet:K_Factor" {
          n247 = Build Array("EnFlo_Tunnel:Pressure:Static", "EnFlo_Tunnel:Reference:Velocity", "Froude:NPL:Atmos_Press", "EnFlo_Tunnel:Temp:Inlet_Av") -> (w727:string[])
          n248 = call "Read_Earlier_Channels.vi"("Present scan array"=w723, "Ch names"=w724, "Desired Channels"=w727) -> ("Scan comments"=w722:string, "Index 0"=w717:dbl, "Index 1"=w714:dbl, "Index 2"=w718:dbl, "Index 3"=w719:dbl)  [unwired: 1 out]
          n249 = Greater?(x=w714, y=0.8) -> (0:w715:bool)
          n250 = case shown="True" w715 {
            tunnel: w719 -> [_ w733]
            tunnel: w718 -> [_ w732]
            tunnel: w714 -> [_ w731]
            tunnel: w717 -> [_ w730]
            tunnel: [nan w729] -> w716
            frame False {
            }
            frame True {
              n251 = formula code="Rho=(Patmos*100)/(287*(T+273));\nDyn_Pres=0.5*Rho*U*U;\nK=(-Pstatic/Dyn_Pres)-1;"("Pstatic"=w730, "Patmos"=w732, "T"=w733, "U"=w731) -> ("K"=w729:dbl)  [unwired: 2 out]
            }
          }
        }
        frame "EnFlo_Tunnel:Chilled Water:Valve Dem Pos" {
          n252 = Get Date/Time In Seconds() -> (seconds since 1Jan1904=w735:timestamp)
          n253 = Concatenate Strings(w736, " last updated") -> (w744:string)
          n254 = To Double Precision Float(number=w735) -> (double precision float=w734:dbl)
          n255 = Unbundle By Name(w742) -> ("A"=w741:dbl)
          n256 = call "Remember_value.vi"("Mode"=Remember_value_mode."Read only", "Ch name"=w744) -> ("Output Value"=w743:dbl)  [unwired: 1 in]
          n257 = Subtract(x=w734, y=w743) -> (x-y=w740:dbl)
          n258 = Greater?(x=w740, y=w741) -> (0:w739:bool)
          n259 = Not A Number/Path/Refnum?(number/path/refnum=w740) -> (NaN/Path/Refnum?=w738:bool)
          n260 = Or(x=w738, y=w739) -> (x .or. y?=w737:bool)
          n261 = case shown="True" w737 {
            tunnel: w751 -> [w752 _]
            tunnel: [w752 w770] -> w750
            tunnel: w749 -> [_ w762]
            tunnel: w748 -> [_ w763]
            tunnel: ["" w768] -> w747
            tunnel: w744 -> [_ w758]
            tunnel: w734 -> [_ w754]
            frame False {
            }
            frame True {
              n262 = call "Read_value_of_earlier_Ch.vi"("Desired Ch to Read"="EnFlo_Tunnel:Chiller_Pump:Enable", "Ch names"=w763, "Present scan array"=w762) -> ("Value"=w761:dbl)  [unwired: 1 in, 1 out]
              n263 = Build Array("EnFlo_Tunnel:Chilled Water:Dem Temp", "EnFlo_Tunnel:Chilled Water:Supply", "EnFlo_Tunnel:Chiller_Pump:Running") -> (w769:string[])
              n264 = call "Read_Earlier_Channels.vi"("Present scan array"=w762, "Ch names"=w763, "Desired Channels"=w769) -> ("Scan comments"=w768:string, "Index 0"=w767:dbl, "Index 1"=w766:dbl, "Index 2"=w756:dbl)  [unwired: 2 out]
              n265 = Greater?(x=w761, y=0.5) -> (0:w759:bool)
              n266 = Greater?(x=w756, y=0.5) -> (0:w755:bool)
              n267 = case shown="True" w755 {
                tunnel: [w785 w792] -> w770
                tunnel: w767 -> [_ w794]
                tunnel: w766 -> [_ w793]
                tunnel: w754 -> [_ w791]
                tunnel: w759 -> [w776 _]
                tunnel: w758 -> [_ w790]
                frame False {
                  n268 = Seconds To Date/Time() -> (date time rec=w773:T14)  [unwired: 2 out]
                  n269 = Unbundle By Name(w773) -> ("day of week"=w780:i32, "hour"=w782:i32)
                  n270 = Less?(x=w782, y=3) -> (x < y?=w777:bool)
                  n271 = Equal?(x=7, y=w780) -> (x = y?=w778:bool)
                  n272 = And(x=w778, y=w777) -> (x .and. y?=w775:bool)
                  n273 = case shown="True" w776 {
                    tunnel: w775 -> [w786 w788]
                    tunnel: [w786 w787] -> w774
                    frame False {
                    }
                    frame True {
                      n274 = Not(x=w788) -> (.not. x?=w787:bool)
                    }
                  }
                  n275 = Select(t=0.0, s=w774, f=100.0) -> (s? t:f=w785:dbl)
                }
                frame True {
                  w796 = 100.0  # Max
                  w797 = 0.0  # Min
                  n276 = call "PID.vi"("Present Value"=w793, "Setpoint"=w794) -> ("Dem Output"=w795:dbl)  [unwired: 1 in]
                  n277 = In Range and Coerce(upper limit=w796, x=w795, lower limit=w797) -> (coerced(x)=w792:dbl)  [unwired: 1 out]
                  n278 = call "Remember_value.vi"("Mode"=Remember_value_mode."Read and Write", "Input Value"=w791, "Ch name"=w790) -> ()  [unwired: 1 out]
                }
              }
            }
          }
        }
        frame "EnFlo_Tunnel:Hydrosonic:Integral" {
          n279 = Build Array("EnFlo_Tunnel:Usonic Fixed:Velocity", "Hydrosonic:Transducer:Setting") -> (w807:string[])
          n280 = call "Read_Earlier_Channels.vi"("Present scan array"=w808, "Ch names"=w806, "Desired Channels"=w807) -> ("Scan comments"=w800:string, "Index 0"=w805:dbl, "Index 1"=w799:dbl)  [unwired: 3 out]
          n281 = Greater?(x=w805, y=0.5) -> (0:w803:bool)
          n282 = case shown="True" w803 {
            tunnel: w802 -> [w811 w819]
            tunnel: [w811 w818] -> w801
            tunnel: w799 -> [_ w817]
            tunnel: w798 -> [_ w816]
            frame False {
            }
            frame True {
              w814 = 8640000.0  # Seconds per day x 100
              n283 = Multiply(x=w817, y=w816) -> (x*y=w815:dbl)
              n284 = Divide(x=w815, y=w814) -> (x/y=w813:dbl)
              n285 = Not A Number/Path/Refnum?(number/path/refnum=w813) -> (NaN/Path/Refnum?=w812:bool)
              n286 = case shown="False" w812 {
                tunnel: w819 -> [w822 w823]
                tunnel: [w821 w823] -> w818
                tunnel: w813 -> [w820 _]
                frame False {
                  n287 = Add(x=w820, y=w822) -> (x+y=w821:dbl)
                }
                frame True {
                }
              }
            }
          }
        }
        frame "EnFlo_Tunnel:Days Run at:2.5m/s" {
          n288 = Build Array("EnFlo_Tunnel:Usonic Fixed:Velocity") -> (w832:string[])
          n289 = call "Read_Earlier_Channels.vi"("Present scan array"=w833, "Ch names"=w831, "Desired Channels"=w832) -> ("Scan comments"=w826:string, "Index 0"=w824:dbl)  [unwired: 4 out]
          n290 = Greater?(x=w824, y=0.5) -> (0:w829:bool)
          n291 = case shown="True" w829 {
            tunnel: w828 -> [w835 w843]
            tunnel: [w835 w842] -> w827
            tunnel: w824 -> [_ w841]
            tunnel: w825 -> [_ w840]
            frame False {
            }
            frame True {
              w838 = 216000.0  # Seconds per day x 2.5
              n292 = Multiply(x=w841, y=w840) -> (x*y=w839:dbl)
              n293 = Divide(x=w839, y=w838) -> (x/y=w837:dbl)
              n294 = Not A Number/Path/Refnum?(number/path/refnum=w837) -> (NaN/Path/Refnum?=w836:bool)
              n295 = case shown="True" w836 {
                tunnel: w843 -> [w846 w847]
                tunnel: [w845 w847] -> w842
                tunnel: w837 -> [w844 _]
                frame False {
                  n296 = Add(x=w844, y=w846) -> (x+y=w845:dbl)
                }
                frame True {
                }
              }
            }
          }
        }
        frame "Complete:Scan:Period" {
          n297 = while {
            tunnel: [w857] -> w850
            tunnel: [w864] -> w852
            shift-left: _ -> [w864]
            shift-right: [w865] -> w853
            tunnel: w849 -> [w861]
            tunnel: [w856] -> w848
            stop <- FALSE continue-if-true
            w856 = 10.0 ("Averaging time (mins)")
            n298 = Build Array(w861) -> (w860:string[])
            n299 = call "Get_Channel_averages.vi"("Desired Ch Names"=w860, "Averaging time (mins)"=w856) -> ("number"=w859:dbl[])  [unwired: 1 in, 2 out]
            n300 = Index Array(array=w859, index=0) -> (element=w857:dbl)
            n301 = Greater?(x=w857, y=20.0) -> (0:w865:bool)
          }
          n302 = Compound Arithmetic op=AND(w853, invert w852) -> (w851:bool)
          n303 = case shown="True" w851 {
            tunnel: w850 -> [_ w871]
            tunnel: w848 -> [_ w866]
            frame False {
            }
            frame True {
              n304 = Format Into String(format string="Warning! The average scan period on the ADAM Scan table is %.1f seconds over the last %d minutes." ("Format String"), w871, w866) -> (resulting string=w869:string)  [unwired: 2 in, 1 out]
              n305 = call "Server_Emails.vi"("Message"=w869, "Contact All clients?"=TRUE, "Subject"="Scan Period") -> ()  [unwired: 2 in, 3 out]
            }
          }
        }
        frame "GMU:Source:Est Time" {
          # "NaN's"
          # "Est?"
          # "Inband?"
          n306 = stacked-sequence {
            seq-local: [w878 _ _ _] -> [_ _ w925 _]
            seq-local: [_ w890 _ _] -> [_ _ w922 _]
            seq-local: [_ w891 _ _] -> [_ _ w920 _]
            seq-local: [_ _ w927 _] -> [_ _ _ w943]
            seq-local: [w882 _ _ _] -> [_ _ w924 _]
            seq-local: [_ w889 _ _] -> [_ _ _ w939]
            tunnel: w877 -> [w884 w892 w930 _]
            tunnel: w876 -> [w883 w893 w931 _]
            tunnel: [_ _ w923 _] -> w875
            tunnel: [_ _ _ w942] -> w874
            tunnel: w873 -> [_ _ _ w941]
            tunnel: w872 -> [_ _ _ w940]
            frame #0 {
              n307 = Build Array("GMU:Source:Density Ratio", "GMU:Source:Dem Strength", "GMU:Source:Dem Q") -> (w885:string[])
              n308 = call "Read_Earlier_Channels.vi"("Present scan array"=w883, "Ch names"=w884, "Desired Channels"=w885) -> ("Scan comments"=w882:string, "Index 0"=w881:dbl, "Index 1"=w880:dbl, "Index 2"=w879:dbl)  [unwired: 2 out]
              n309 = Build Array(w881, w880, w879) -> (w878:dbl[])
            }
            frame #1 {
              n310 = for {
                N: 2 -> [_]
                tunnel: w893 -> [w903]
                tunnel: w892 -> [w904]
                tunnel: [w902] -> w890 mode=indexing
                tunnel: [w909] -> w891 mode=indexing
                tunnel: [w908] -> w889 mode=indexing
                i -> [w914]
                w913 = 23.0  # %
                n311 = case shown="1" w914 {
                  tunnel: ["GMU:Source:Meas Q" "GMU:Source:Meas Strength"] -> w907
                  tunnel: ["GMU:Source:Dem Q" "GMU:Source:Dem Strength"] -> w906
                  frame 0, Default {
                  }
                  frame 1 {
                  }
                }
                n312 = Build Array(w906, w907) -> (w905:string[])
                n313 = call "Read_Earlier_Channels.vi"("Present scan array"=w903, "Ch names"=w904, "Desired Channels"=w905) -> ("Scan comments"=w902:string, "Index 0"=w900:dbl, "Index 1"=w901:dbl)  [unwired: 3 out]
                n314 = Not A Number/Path/Refnum?(number/path/refnum=w901) -> (NaN/Path/Refnum?=w908:bool)
                n315 = Subtract(x=w901, y=w900) -> (x-y=w899:dbl)
                n316 = Greater Than 0?(x=w900) -> (x > 0?=w910:bool)
                n317 = Less?(x=w899, y=0.05) -> (x < y?=w896:bool)
                n318 = call "In_Range_check.vi"("%"=w913, "Mode"=In_Range."%", "Value"=w901, "Setpoint"=w900) -> ("In Range"=w897:bool)  [unwired: 1 in, 2 out]
                n319 = Or(x=w897, y=w896) -> (x .or. y?=w895:bool)
                n320 = And(x=w895, y=w910) -> (x .and. y?=w911:bool)
                n321 = Compound Arithmetic op=OR(w911, invert w910, w908) -> (w909:bool)
              }
            }
            frame #2 {
              n322 = while {
                tunnel: [w938] -> w926
                tunnel: w925 -> [w937]
                shift-left: _ -> [w938]
                shift-right: [w937] -> _
                stop <- FALSE continue-if-true
              }
              n323 = Equal?(x=w925, y=w926) -> (x = y?=w932:bool)
              n324 = call "Read_value_of_earlier_Ch.vi"("Desired Ch to Read"="GMU:Source:Dem Q", "Ch names"=w930, "Present scan array"=w931) -> ("Value"=w928:dbl)  [unwired: 1 in, 1 out]
              n325 = Greater Than 0?(x=w928) -> (x > 0?=w935:bool)
              n326 = And Array Elements(Boolean array=w920) -> (logical AND=w919:bool)
              n327 = Select(t=w919, s=w935, f=TRUE) -> (s? t:f=w933:bool)
              n328 = Compound Arithmetic op=AND(w932, w933) -> (w927:bool)
              n329 = Concatenate Strings(w922) -> (w921:string)
              n330 = Concatenate Strings(w921, w924) -> (w923:string)
            }
            frame #3 {
              n331 = case shown="True" w943 {
                tunnel: [0.0 w945] -> w942
                tunnel: w941 -> [_ w950]
                tunnel: w940 -> [_ w946]
                tunnel: w939 -> [_ w949]
                frame False {
                }
                frame True {
                  n332 = Or Array Elements(Boolean array=w949) -> (logical OR=w948:bool)
                  n333 = Add(x=w950, y=w946) -> (x+y=w947:dbl)
                  n334 = Select(t=w946, s=w948, f=w947) -> (s? t:f=w945:dbl)
                }
              }
            }
          }
        }
      }
    }
    frame "Hold Value" {
    }
    frame "Read A" {
      n335 = Unbundle By Name(w954) -> ("A"=w953:dbl)
    }
    frame "Read Ch" {
      n336 = Unbundle By Name(w959) -> ("String"=w956:string)
      n337 = call "Read_value_of_earlier_Ch.vi"("Desired Ch to Read"=w956, "Ch names"=w960, "Present scan array"=w961) -> ("Value"=w957:dbl, "Scan comment"=w958:string)  [unwired: 1 in]
    }
    frame "Coded" {
    }
    frame "Client Info" {
      n338 = global read "ADAM_Global.vi" "Client State Array"() -> (w976:T15[])
      n339 = call "Split_Ch_name.vi"("Ch name"=w970) -> ("Top level"=w968:string, "Low level"=w966:string)  [unwired: 1 out]
      n340 = Equal?(x="Status" ("Substring"), y=w968) -> (x = y?=w967:bool)
      n341 = Select(t=w966, s=w967, f="") -> (s? t:f=w964:string)
      n342 = for {
        tunnel: w976 -> [w985] mode=indexing
        tunnel: [w984] -> w977 mode=indexing
        n343 = Unbundle By Name(w985) -> ("Client Name"=w984:string)
      }
      n344 = Search 1D Array(1D array=w977, element=w964) -> (index of element=w972:i32)  [unwired: 1 out]
      n345 = Less Than 0?(x=w972) -> (x < 0?=w971:bool)
      n346 = Index Array(array=w976, index=w972) -> (element=w975:T15)
      n347 = case shown="False" w971 {
        tunnel: w975 -> [w980 _]
        tunnel: w964 -> [w979 w982]
        tunnel: [w978 w981] -> w974
        frame False {
          n348 = call "Get_Client_Status_string.vi"("Client State Cluster"=w980, "Client Name"=w979) -> ("Code Value"=w978:dbl)  [unwired: 1 in]
        }
        frame True {
          w981 = 7.0 ("Code Value")
          n349 = call "Remember_value.vi"("Mode"=Remember_value_mode."Read and Write", "Input Value"=w981, "Ch name"=w982) -> ()  [unwired: 1 out]
        }
      }
    }
    frame "Web Client" {
      w995 = 7200.0  # 2 Hours in Seconds
      n350 = Concatenate Strings(w1004, ":Last read" ("Substring")) -> (w1002:string)
      n351 = call "Remember_value.vi"("Mode"=Remember_value_mode."Read only", "Ch name"=w1002) -> ("Output Value"=w1001:dbl)  [unwired: 1 in]
      n352 = Not A Number/Path/Refnum?(number/path/refnum=w1001) -> (NaN/Path/Refnum?=w999:bool)
      n353 = Get Date/Time In Seconds() -> (seconds since 1Jan1904=w994:timestamp)
      n354 = To Double Precision Float(number=w994) -> (double precision float=w992:dbl)
      n355 = Subtract(x=w992, y=w1001) -> (x-y=w1007:dbl)
      n356 = Greater?(x=w1007, y=1800.0) -> (0:w1000:bool)
      n357 = Or(x=w1000, y=w999) -> (x .or. y?=w986:bool)
      n358 = case shown="True" w986 {
        frame False {
        }
        frame True {
          n359 = global read "Constants_global.vi" "EnFlo SW Folder"() -> (w1010:path)
          n360 = Build Path(base path=w1010, name or relative path=path "ADAM Server/Sub VI's/Web_Client.vi") -> (appended path=w1009:path)
          n361 = Open VI Reference(vi path=w1009) -> (vi reference=w1014:refnum<vi>, error out=w1015:errorcluster)  [unwired: 1 in, 4 out]
          n362 = property class="VI"(reference=w1014, error in=w1015) -> (reference out=w1017:refnum<vi>, error out=w1018:errorcluster, "Front Panel Window:Open"=w1016:bool)
          n363 = case shown="False" w1016 {
            tunnel: w1017 -> [w1024 w1027]
            tunnel: w1018 -> [w1023 w1026]
            tunnel: [w1022 w1027] -> w1019
            tunnel: [w1021 w1026] -> w1020
            frame False {
              n364 = property class="VI"(reference=w1024, error in=w1023, "Front Panel Window:Open"=TRUE) -> (reference out=w1022:refnum<vi>, error out=w1021:errorcluster)
            }
            frame True {
            }
          }
          n365 = invoke class="VI" method="Run VI"(reference=w1019, error in=w1020, "Wait until done"=FALSE, "Auto Dispose Ref"=TRUE) -> ()  [unwired: 1 in, 5 out]
        }
      }
      n366 = Concatenate Strings(w1004, ":value time" ("Substring")) -> (w988:string)
      n367 = call "Remember_value.vi"("Mode"=Remember_value_mode."Read only", "Ch name"=w1004) -> ("Output Value"=w1008:dbl)  [unwired: 1 in]
      n368 = call "Remember_value.vi"("Mode"=Remember_value_mode."Read only", "Ch name"=w988) -> ("Output Value"=w993:dbl)  [unwired: 1 in]
      n369 = Subtract(x=w992, y=w993) -> (x-y=w991:dbl)
      n370 = Greater?(x=w991, y=w995) -> (0:w998:bool)
      n371 = case shown="True" w998 {
        tunnel: w991 -> [_ w1033]
        tunnel: 3600.0 ("y") -> [_ w1032]
        tunnel: ["" w1030] -> w997
        frame False {
        }
        frame True {
          n372 = Divide(x=w1033, y=w1032) -> (x/y=w1029:dbl)
          n373 = Format Into String(format string="Value is %d hours old." ("Format String"), w1029) -> (resulting string=w1030:string)  [unwired: 2 in, 1 out]
        }
      }
    }
    frame "X10" {
      (unwired) 1 items=["-----", "A", "B", "C", "D", "E", "F", "G", "H", "I", "J", "K", "L", "M", "N", "O", "P"] ("House Code")
      n374 = Greater Than 0?(x=w1038) -> (x > 0?=w1037:bool)
      n375 = Unbundle By Name(w1043) -> ("Port Name"=w1040:string, "Main"=w1041:i32, "Ch."=w1042:i32)
      n376 = call "X10control.vi"("Port Name"=w1040, "Power Request (ON)"=w1037, "House Code"=w1041, "Unit No."=w1042) -> ()  [unwired: 6 out]
      n377 = Select(t=1.0, s=w1037, f=0.0) -> (s? t:f=w1034:dbl)
    }
    frame "LPA" {
      # "LPA was, IIRC, a serially-polled weighing platform we rented at Surrey for Athena Scaperdas' project at Atkins to weigh a helicopter with rotor running. \nTo add to the fun, it was RS232, so to make it addressable it was polled through an addressable ADAM 485-232 module"
      n378 = call "LPA400_get_rdg.vi"("Channel Name"=w1046, "Address"=w1047) -> ("Output"=w1044:dbl, "Status note"=w1045:string)  [unwired: 4 out]
    }
    frame "ScanPacer" {
      # "Uses a metronome to slow an otherwise over-fast scan table"
      n379 = call "ADAMPacer.vi"("Ch Description"=w1050) -> ("Scan comment"=w1048:string, "Output"=w1049:dbl)  [unwired: 7 in]
    }
    frame "Test" {
      w1054 = 0.0005  # y
      n380 = Get Date/Time In Seconds() -> (seconds since 1Jan1904=w1051:timestamp)
      n381 = To Double Precision Float(number=w1051) -> (double precision float=w1056:dbl)
      n382 = Subtract(x=w1056, y=2969882881.0) -> (x-y=w1055:dbl)
      n383 = Multiply(x=w1055, y=w1054) -> (x*y=w1052:dbl)
      n384 = Random Number (0-1)() -> (number: 0 to 1=w1053:dbl)
      n385 = Add(x=w1053, y=w1052) -> (x+y=w1059:dbl)
    }
    frame "Oops", Default {
    }
  }
  "Output" <- w8
  "Scan comment" <- w5
